vi "moveComplete-Event.vi"(8 "Error In":errorcluster) -> (0 "Error Out":errorcluster)   [LabVIEW 2016]
doc: "André Romero - 2023\nandretec@ifsc.usp.br\nIFSC - USP"
uses:
  Global Motors.vi
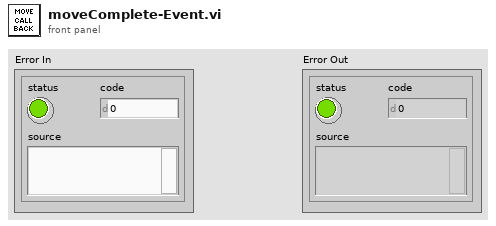
[diagram p1: front panel]
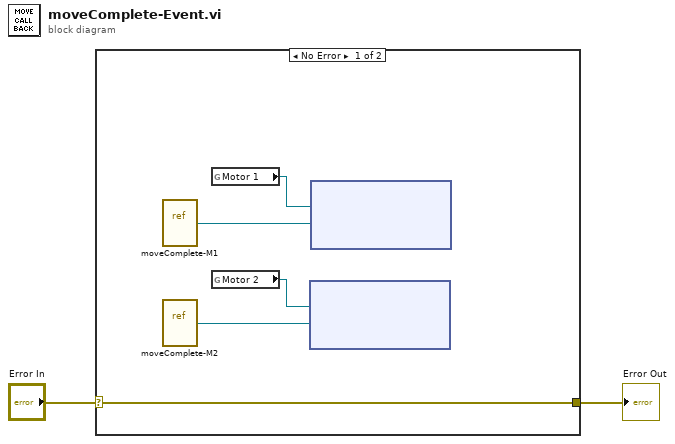
[diagram p0: block diagram]
diagram:
  n1 = case shown="No Error" "Error In" {
    selector: "Error In" -> [w3 w8]
    tunnel: [w3 w8] -> w1
    frame No Error {
      n2 = vi-ref "moveComplete-M1.vi"() -> ("vi reference"=w7:refnum<vi>)
      n3 = vi-ref "moveComplete-M2.vi"() -> ("vi reference"=w6:refnum<vi>)
      n4 = global read "Global Motors.vi" "Motor 1"() -> (w5:refnum<k7>)
      n5 = global read "Global Motors.vi" "Motor 2"() -> (w4:refnum<k7>)
      n6 = node(w4, w6) -> ()  [unwired: 3 in, 2 out]
      n7 = node(w5, w7) -> ()  [unwired: 3 in, 2 out]
    }
    frame Error {
    }
  }
  "Error Out" <- w1
